vi "Stop Widget Engine.vi"(8 "Error In":errorcluster) -> (0 "Error Out":errorcluster)   [LabVIEW 2013, in "Template.lvlib" / "LQWidgetEngine.lvclass"]
uses:
  LQWidgetEngine.lvclass
  Private/Global Quit Event Holder.vi
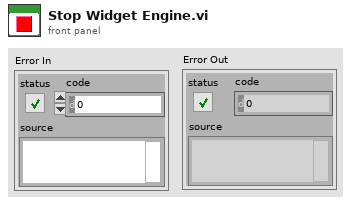
[diagram p1: front panel]
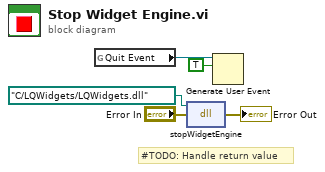
[diagram p0: block diagram]
diagram:
  # "#TODO: Handle return value"
  n1 = global read "Global Quit Event Holder.vi" "Quit Event"() -> (w2:refnum<user-event>)
  n2 = dll-call lib="?" fn="stopWidgetEngine"(path in=path "C:/LQWidgets/LQWidgets.dll", error in="Error In") -> (error out=→"Error Out":errorcluster)  [unwired: 2 in, 1 out]
  n3 = Generate User Event(user event=w2, event data cluster=TRUE ("event data")) -> ()  [unwired: 2 in, 2 out]
